vi "set_value_REF.vi"(5 "treat value as XML?":bool, 7 "attribute name":string, 8 "error in (no error)":errorcluster, 10 "value":string, 11 "Element ref in":refnum<k20>) -> (0 "error out":errorcluster, 3 "Element ref out":refnum<k20>)   [LabVIEW 2010, in "XMLElement.lvclass"]
uses:
  XMLElement.lvclass
  Program Files (x86)/National Instruments/LabVIEW 2010/resource/objmgr/DOMUserDefRef.rc
  <vilib>/xml/NI_XML.lvlib
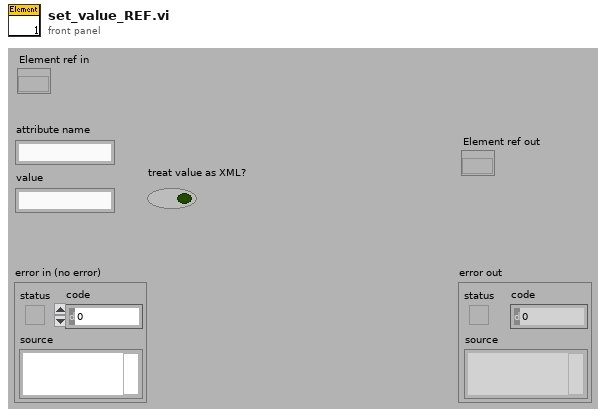
[diagram p1: front panel]
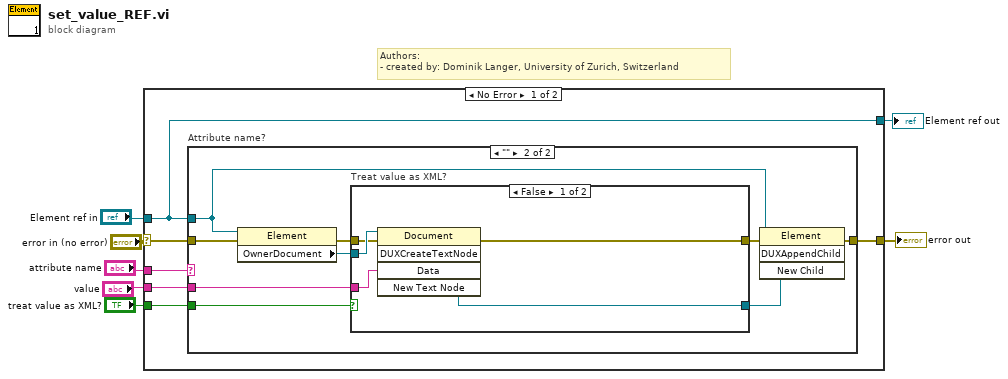
[diagram p0: block diagram]
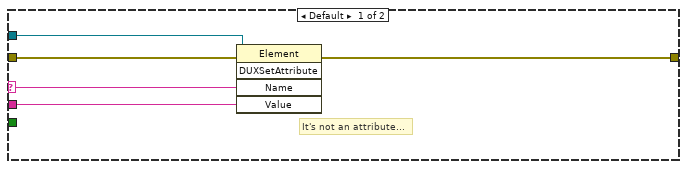
[diagram p2: hidden frame]
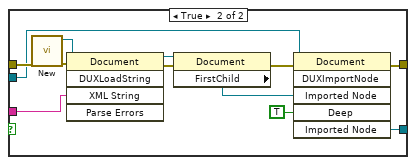
[diagram p3: hidden frame]
diagram:
  # "Authors: \n- created by: Dominik Langer, University of Zurich, Switzerland"
  n1 = case shown="No Error" "error in (no error)" {
    selector: "error in (no error)" -> [w13 w46]
    tunnel: [w12 w46] -> w6
    tunnel: "value" -> [w11 _]
    tunnel: "attribute name" -> [w10 _]
    tunnel: "Element ref in" -> [w9 w45]
    tunnel: [w9 w45] -> w2
    tunnel: "treat value as XML?" -> [w8 _]
    frame No Error {
      n2 = case "Attribute name?" shown="\"\"" w10 {
        selector: w10 -> [w14 _]
        tunnel: w9 -> [w18 w20]
        tunnel: w13 -> [w17 w22]
        tunnel: w11 -> [w16 w25]
        tunnel: [w15 w26] -> w12
        tunnel: w8 -> [_ w24]
        frame Default {
          # "It's not an attribute..."
          n3 = invoke class="Element" method="DUXSetAttribute"(reference=w18, error in=w17, "Name"=w14, "Value"=w16) -> (error out=w15:errorcluster)  [unwired: 1 in, 4 out]
        }
        frame "" {
          n4 = property class="Element"(reference=w20, error in=w22) -> (error out=w21:errorcluster, "OwnerDocument"=w19:refnum<k20>)  [unwired: 1 out]
          n5 = case "Treat value as XML?" shown="False" w24 {
            tunnel: [w32 w37] -> w27
            tunnel: w21 -> [w28 w41]
            tunnel: w25 -> [w31 w39]
            tunnel: [w30 w34] -> w23
            tunnel: w19 -> [w29 w36]
            frame False {
              n6 = invoke class="Document" method="DUXCreateTextNode"(reference=w29, error in=w28, "Data"=w31) -> (error out=w32:errorcluster, "New Text Node"=w30:refnum<k20>)  [unwired: 2 in, 3 out]
            }
            frame True {
              n7 = call <vilib>:"New.vi"("error in (no error)"=w41) -> ("error out"=w43:errorcluster, "DOM document out"=w40:refnum<k20>)  [unwired: 7 in]
              n8 = invoke class="Document" method="DUXLoadString"(reference=w40, error in=w43, "XML String"=w39) -> (reference out=w42:refnum<k20>, error out=w44:errorcluster)  [unwired: 2 in, 3 out]
              n9 = property class="Document"(reference=w42, error in=w44) -> (error out=w38:errorcluster, "FirstChild"=w35:refnum<k20>)  [unwired: 1 out]
              n10 = invoke class="Document" method="DUXImportNode"(reference=w36, error in=w38, "Imported Node"=w35, "Deep"=TRUE) -> (error out=w37:errorcluster, "Imported Node"=w34:refnum<k20>)  [unwired: 2 in, 4 out]
            }
          }
          n11 = invoke class="Element" method="DUXAppendChild"(reference=w20, error in=w27, "New Child"=w23) -> (error out=w26:errorcluster)  [unwired: 1 in, 3 out]
        }
      }
    }
    frame Error {
    }
  }
  "error out" <- w6
  "Element ref out" <- w2
